vi "Clear.vi"(8 "error in (no error)":errorcluster, 11 "Mock Data Listener in":refnum<class "Mock Data Listener.lvclass">) -> (0 "error out":errorcluster)   [LabVIEW 2020, in "Mock Data Listener.lvclass"]
uses:
  Mock Data Listener.lvclass
  Mock Data Listener.lvclass/Mock Data Listener.ctl
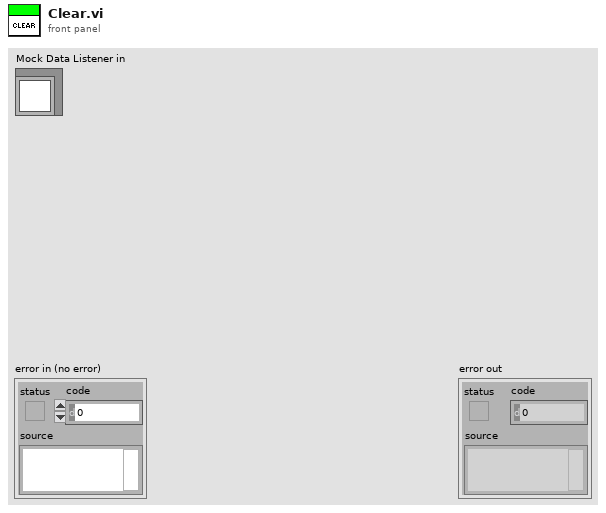
[diagram p1: front panel]
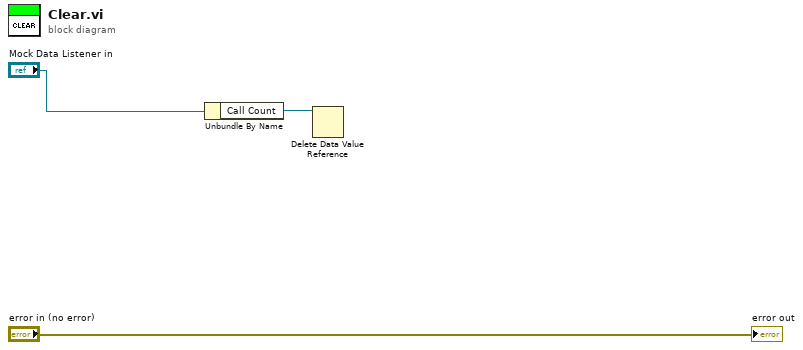
[diagram p0: block diagram]
diagram:
  n1 = Unbundle By Name("Mock Data Listener in") -> ("Call Count"=w1:refnum<data-value>)
  n2 = Delete Data Value Reference(data value reference=w1) -> ()  [unwired: 1 in, 2 out]
  "error out" <- "error in (no error)"
